vi "oa_FIR Preprocess Filter Linear to dB.vi"(1 "linear value":dbl) -> (0 "dB value":dbl)   [LabVIEW 2017, in "SoundVib_RefDataProcess.lvlib"]
uses:
  <vilib>/addons/Sound and Vibration/Order Analysis/Referece Data Processing/SoundVib_RefDataProcess.lvlib
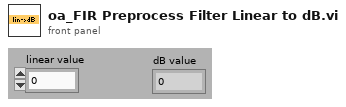
[diagram p1: front panel]
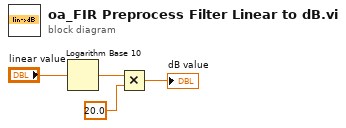
[diagram p0: block diagram]
diagram:
  n1 = Logarithm Base 10(1:"linear value") -> (0:w3:dbl)
  n2 = Multiply(x=w3, y=20.0) -> (x*y=→"dB value":dbl)
